vi "GetCompletedFrame_DEPRECATED.vi"(8 "error in (no error)":errorcluster, 10 "ActualBufferNumber":u32, 11 "reference in":refnum<class "Camera_IMAQdx.lvclass">) -> (0 "error out":errorcluster, 1 "Frame Number":u32, 2 "Image Out":T1, 3 "reference out":refnum<class "Camera_IMAQdx.lvclass">)   [LabVIEW 2017]
doc: "Gets the frame that was just completed from the acquisition buffer. This is to be called when the Frame Complete event is fired."
uses:
  Camera_IMAQdx.lvclass
  <vilib>/vision/driver/NI_Vision_Acquisition_Software.lvlib
  <vilib>/vision/driver/IMAQdx.llb/IMAQdx Buffer Number Mode.ctl
  <vilib>/vision/Image Controls.llb/IMAQ Image.ctl
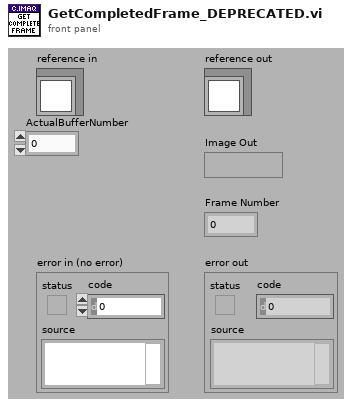
[diagram p1: front panel]
types:
  T1 = typedef "IMAQ Image.ctl" = refnum<image>
  T2 = typedef "NI_Vision_Acquisition_Software.lvlib/IMAQdx Buffer Number Mode.ctl" = enum32{"Next", "Last", "Buffer Number", "Every", "Last New"}
  T3 = typedef "IMAQdx.ctl" = refnum<k21>
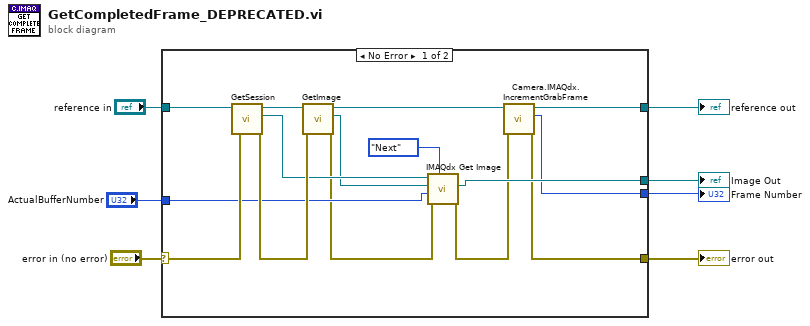
[diagram p0: block diagram]
diagram:
  n1 = case shown="No Error" "error in (no error)" {
    selector: "error in (no error)" -> [w19 w24]
    tunnel: [w8 w24] -> w6
    tunnel: [w11 w23] -> w4
    tunnel: "reference in" -> [w18 w23]
    tunnel: [w14 _] -> w2
    tunnel: [w10 _] -> w3
    tunnel: "ActualBufferNumber" -> [w15 _]
    frame No Error {
      n2 = call "GetSession.vi"("error in (no error)"=w19, "reference in"=w18) -> ("error out"=w21:errorcluster, "Session"=w17:T3, "reference out"=w22:refnum<class "Camera_IMAQdx.lvclass">)  [unwired: 7 in]
      n3 = call "GetImage.vi"("error in (no error)"=w21, "reference in"=w22) -> ("error out"=w13:errorcluster, "Image"=w16:T1, "reference out"=w20:refnum<class "Camera_IMAQdx.lvclass">)  [unwired: 7 in]
      n4 = call <vilib>:"IMAQdx Get Image.vi"("Buffer Number Mode (Next)"=IMAQdx_Buffer_Number_Mode."Next", "error in"=w13, "Buffer Number In"=w15, "Image In"=w16, "Session In"=w17) -> ("error out"=w9:errorcluster, "Image Out"=w14:T1)  [unwired: 3 in, 2 out]
      n5 = call "Camera.IMAQdx.IncrementGrabFrame.vi"("error in (no error)"=w9, "reference in"=w20) -> ("error out"=w8:errorcluster, "Frame Number"=w10:u32, "reference out"=w11:refnum<class "Camera_IMAQdx.lvclass">)  [unwired: 7 in]
    }
    frame Error {
    }
  }
  "error out" <- w6
  "reference out" <- w4
  "Image Out" <- w2
  "Frame Number" <- w3
